vi "IR test 002.vi"() -> ()   [LabVIEW 2019]
uses:
  low level/IR sensor/IR sensor.lvclass
panel:
  out "IR":dbl
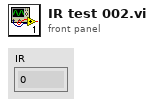
[diagram p1: front panel]
types:
  T1 = enum16{"IR.1", "IR.2", "IR.3", "IR.4", "IR.5", "IR.6", "IR.7", "IR.8"}
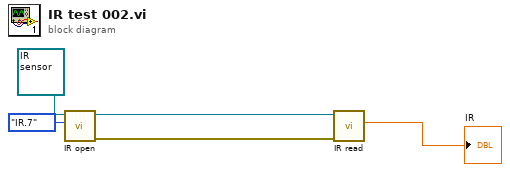
[diagram p0: block diagram]
diagram:
  n1 = call-dynamic "IR open.vi"("IR pin"=T1."IR.7", "IR sensor in"=refnum<class "IR sensor.lvclass"> refnum) -> ("error out"=w4:errorcluster, "IR sensor out"=w5:refnum<class "IR sensor.lvclass">)  [unwired: 8 in]
  n2 = call-dynamic "IR read.vi"("error in (no error)"=w4, "IR sensor in"=w5) -> ("IR"=→"IR":dbl)  [unwired: 7 in, 2 out]
